vi "Send PCP return data to processing.vi"(1 "PCP Action":T1, 5 "Return Data":variant, 11 "error in":errorcluster, 12 "Reply Received":bool, 13 "Reply Expected":bool) -> (15 "error out":errorcluster)   [LabVIEW 2011]
uses:
  PCP Commands.ctl
  PCP Command Return.ctl
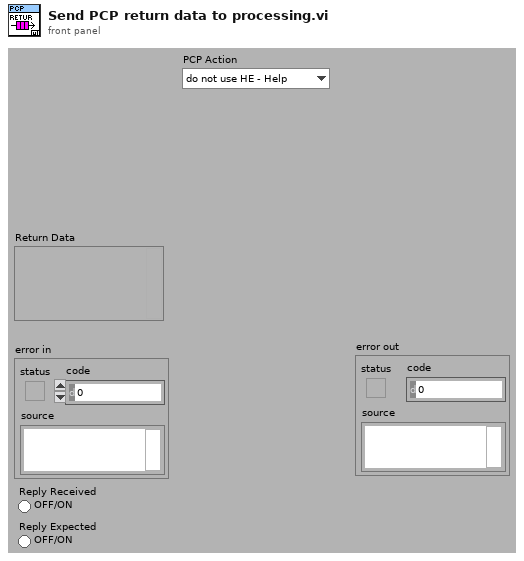
[diagram p1: front panel]
types:
  T1 = typedef "PCP Commands.ctl" = enum16{"do not use HE - Help", "RDd - Most used inputs", "RA - All analog inputs", "RE n Reset DO n", "SE n Set DO n", "RP - Get digital inputs", "VA d Set AO A  Motor Volt", "VB d Set AO B  Cable Resistance", "VEr - Get Version", "DYp - Depth counter", "DR - Reset Depth Counter", "DS n Set Depth options(0-3)", "do not use ME - Manual mode enabled", "MD - Manual mode disabled", "ID - Get ID(2001)", "TS - Get Timestamp", "TO d(s)  Set timeout", "do not use LO n Start Loop Mode(1,2)", "AL n RD&LO variation", "ST - Stop Loop Mode"}
  T2 = typedef "PCP Command Return.ctl" = cluster{"Action":T1, "Data in return":variant}
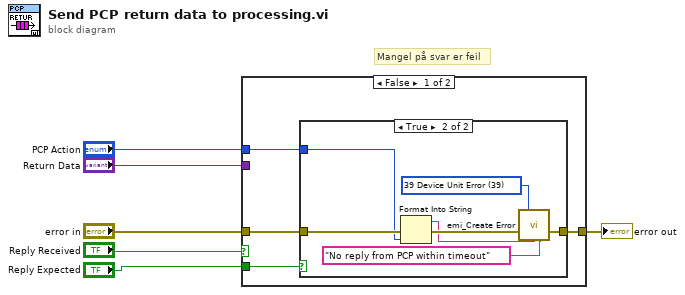
[diagram p0: block diagram]
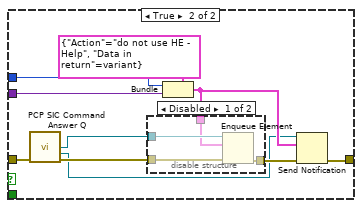
[diagram p3: hidden frame]
diagram:
  # "Mangel på svar er feil"
  n1 = case shown="False" "Reply Received" {
    tunnel: "error in" -> [w9 w24]
    tunnel: "Return Data" -> [_ w26]
    tunnel: "PCP Action" -> [w8 w27]
    tunnel: [w10 w21] -> w6
    tunnel: "Reply Expected" -> [w7 _]
    frame False {
      n2 = case shown="True" w7 {
        tunnel: [w11 w18] -> w10
        tunnel: w9 -> [w11 w15]
        tunnel: w8 -> [_ w13]
        frame False {
        }
        frame True {
          w17 = 39 items=["0 No Error"=0, "1 Invalid input parameter"=1, "6 Generic file IO "=6, "7 File not Found"=7, "35 Generic Pring Error"=35, "37 Device not Found"=37, "39 Device Unit Error"=39, "40 Could fot Open Device"=40, "42 Generic Error"=42, "52 Unknown Message"=52, "98 Bad File type"=98, "99 Bad File Version"=99, "100 Bad Data in File"=100, "1018 Unspecefied Error"=1018, "1041 Incorrect Password"=1041, "1043 Feature not in this version"=1043, "1109 Unsuported Data type"=1109, "1444 Did not close sucessfully"=1444] ("Error Code")
          n3 = Format Into String(error in=w15, w13) -> (resulting string=w12:string, error out=w14:errorcluster)  [unwired: 2 in]
          n4 = call "emi_Create Error.vi"("Error Code"=w17, "error in (no error)"=w14, "Source String(\"\")"=w12, "Append String(\"\")"="No reply from PCP within timeout" ("Source String(\"\")")) -> ("error out"=w18:errorcluster)  [unwired: 11 in]
        }
      }
    }
    frame True {
      n5 = call "PCP SIC Command Answer Q.vi"("error in (no error)"=w24) -> ("PCP Ans Q"=w23:refnum<queue>, "PCP Ans Not"=w19:refnum<notifier>, "error out"=w22:errorcluster)  [unwired: 12 in]
      n6 = Bundle(cluster=T2 {"Action"=enum."do not use HE - Help", "Data in return"=variant} ("PCP command definer"), "Action"=w27, "Data in return"=w26) -> (w20:T2)
      n7 = disable-structure shown="Disabled" {
        disable-tunnel: [w32 w33] -> w25
        disable-tunnel: w23 -> [w31 _]
        disable-tunnel: w22 -> [w30 w33]
        disable-tunnel: w20 -> [w29 _]
        frame Disabled {
          n8 = Enqueue Element(queue=w31, element=w29, error in (no error)=w30) -> (error out=w32:errorcluster)  [unwired: 1 in, 2 out]
        }
        frame Enabled {
        }
      }
      n9 = Send Notification(notification=w20, notifier=w19, error in (no error)=w25) -> (error out=w21:errorcluster)  [unwired: 1 out]
    }
  }
  "error out" <- w6
